vi "Measure dt.vi"() -> (3 "dt":u32)   [LabVIEW 2016, in "SMD-7615.lvlib"]
doc: "Helper VI to measure time in ms between two calls"
uses:
  SMD-7615.lvlib
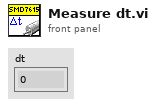
[diagram p1: front panel]
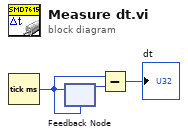
[diagram p0: block diagram]
diagram:
  n1 = Tick Count (ms)() -> (millisecond timer value=w2:u32)
  n2 = feedback #1(w2) -> (w1:u32)
  n3 = feedback-in #1(w2) -> ()
  n4 = Subtract(x=w2, y=w1) -> (x-y=→"dt":u32)
